vi "手动启动选择对话框.vi"() -> (2 "确定":bool, 3 "参数启用":T1)   [LabVIEW 2016, in "PLC.lvlib"]
uses:
  PLC.lvlib
panel:
  in  "CODCr":bool
  in  "总磷总氮":bool
  in  "氨氮":bool
  in  "CODmn":bool
  in  "多参数":bool
  in  "取消":bool
  in  "确定":bool
  # "请选择启动参数"
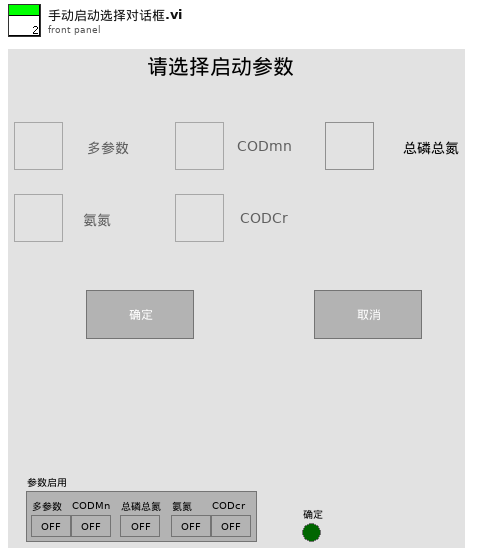
[diagram p1: front panel]
types:
  T1 = cluster{"多参数":bool, "CODMn":bool, "总磷总氮":bool, "氨氮":bool, "CODcr":bool}
  T2 = enum8{"Enabled", "Disabled", "Disabled and Grayed Out"}
  T3 = cluster{"多参数":bool, "CODmn":bool, "总磷总氮":bool, "氨氮":bool, "CODCr":bool}
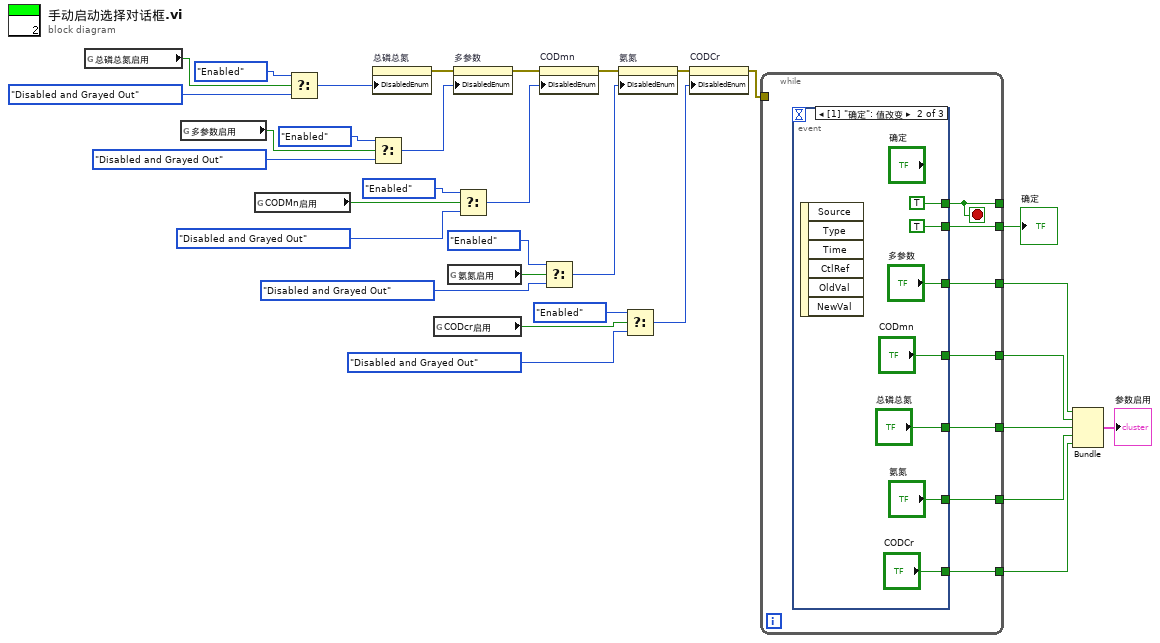
[diagram p0: block diagram]
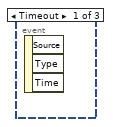
[diagram p2: hidden frame]
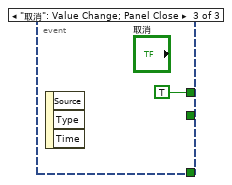
[diagram p3: hidden frame]
diagram:
  n1 = global read "系统设置全局变量.vi" "总磷总氮启用"() -> (w25:bool)
  n2 = global read "系统设置全局变量.vi" "多参数启用"() -> (w7:bool)
  n3 = global read "系统设置全局变量.vi" "CODMn启用"() -> (w11:bool)
  n4 = Select(t=T2."Enabled" ("禁用"), s=w25, f=T2."Disabled and Grayed Out" ("禁用")) -> (s? t:f=w22:T2)
  n5 = property on="总磷总氮" class="Bool (严格)"("DisabledEnum"=w22) -> (error out=w5:errorcluster)  [unwired: 2 in, 1 out]
  n6 = Select(t=T2."Enabled" ("禁用"), s=w7, f=T2."Disabled and Grayed Out" ("禁用")) -> (s? t:f=w6:T2)
  n7 = global read "系统设置全局变量.vi" "CODcr启用"() -> (w9:bool)
  n8 = global read "系统设置全局变量.vi" "氨氮启用"() -> (w13:bool)
  n9 = property on="多参数" class="Bool (严格)"(error in=w5, "DisabledEnum"=w6) -> (error out=w4:errorcluster)  [unwired: 1 in, 1 out]
  n10 = Select(t=T2."Enabled" ("禁用"), s=w11, f=T2."Disabled and Grayed Out" ("禁用")) -> (s? t:f=w10:T2)
  n11 = property on="CODmn" class="Bool (严格)"(error in=w4, "DisabledEnum"=w10) -> (error out=w3:errorcluster)  [unwired: 1 in, 1 out]
  n12 = Select(t=T2."Enabled" ("禁用"), s=w13, f=T2."Disabled and Grayed Out" ("禁用")) -> (s? t:f=w12:T2)
  n13 = property on="氨氮" class="Bool (严格)"(error in=w3, "DisabledEnum"=w12) -> (error out=w2:errorcluster)  [unwired: 1 in, 1 out]
  n14 = Select(t=T2."Enabled" ("禁用"), s=w9, f=T2."Disabled and Grayed Out" ("禁用")) -> (s? t:f=w8:T2)
  n15 = property on="CODCr" class="Bool (严格)"(error in=w2, "DisabledEnum"=w8) -> (error out=w1:errorcluster)  [unwired: 1 in, 1 out]
  n16 = while {
    tunnel: [w39] -> w32
    tunnel: [w38] -> w27
    tunnel: [w37] -> w29
    tunnel: [w36] -> _
    tunnel: [w35] -> w31
    tunnel: [w34] -> w28
    tunnel: [w33] -> w26
    tunnel: w1 -> [_]
    stop <- w36 stop-if-true
    n17 = event shown="[1] \"确定\": 值改变" {
      selector: _ -> [_ _ _]
      dyn-events: _ -> [_ _ _]
      timeout: _ -> [_ _ _]
      tunnel: [_ TRUE TRUE] -> w36
      tunnel: [_ "多参数" _] -> w39
      tunnel: [_ "氨氮" _] -> w38
      tunnel: [_ "CODmn" _] -> w37
      tunnel: [_ TRUE _] -> w35
      tunnel: [_ "总磷总氮" _] -> w34
      tunnel: [_ "CODCr" _] -> w33
      event Timeout {
        n18 = event-data() -> ()  [unwired: 1 in, 3 out]
      }
      event "确定": Value Change {
        n19 = event-data() -> ()  [unwired: 1 in, 6 out]
      }
      event "取消": Value Change; Panel Close {
        n20 = event-data() -> ()  [unwired: 1 in, 3 out]
      }
    }
  }
  "确定" <- w31
  n21 = Bundle("多参数"=w32, "CODmn"=w29, "总磷总氮"=w28, "氨氮"=w27, "CODCr"=w26) -> (→"参数启用":T3)  [unwired: 1 in]
